vi "Entry.vi"(8 "error in (no error)":errorcluster, 11 "New State":refnum<class "Init_cls.lvclass">) -> (0 "error out":errorcluster, 3 "State out":refnum<class "Init_cls.lvclass">)   [LabVIEW 2025, in "Demo_States.lvlib" / "Init_cls.lvclass"]
doc: "This is an abstract method. Override this method to define the behavior when you enter the state."
uses:
  Init_cls.lvclass
  Demo_States/Demo_States.lvclass
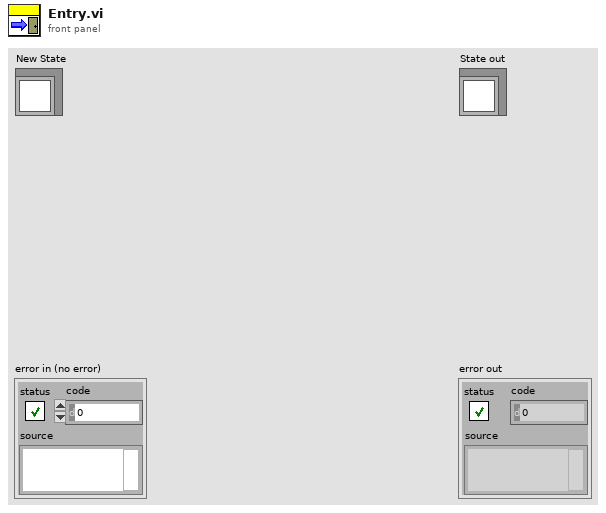
[diagram p1: front panel]
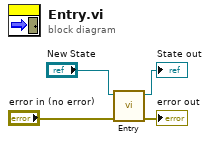
[diagram p0: block diagram]
diagram:
  n1 = call-parent "Entry.vi"("error in (no error)"="error in (no error)", "New State"="New State") -> ("error out"=→"error out":errorcluster, "State out"=→"State out":refnum<class "Init_cls.lvclass">)  [unwired: 8 in]
